vi "RSZVB Select PAE Measurement.vi"(6 "DUT Out (2)":i32=2, 7 "DUT In (1)":i32=1, 8 "error in (no error)":errorcluster {"code" format="%.0x"}, 9 "Trace Name (Trc1)":string="Trc1", 10 "Channel (1)":i32=1, 11 "VISA session":refnum<visa-resource-name>) -> (0 "error out":errorcluster {"code" format="%.0x"}, 3 "dup VISA session":refnum<visa-resource-name>)   [LabVIEW 2011]
doc: "This VI select the Power Added Efficiency (PAE) of an active 2-port device as measured quantity and to define the parameters for the PAE measurement. \n\nThe Power Added Efficiency (PAE) is the ratio of the added RF power generated by an active two-port device (e.g. an amplifier) to the supplied DC power PDC. The added RF power can be expressed as the difference between the power of the outgoing wave b2 at the output of the DUT and the power of the incident wave a1 at the input of the DUT.\n\nAssigns a measurement parameter to an existing trace or creates a trace and assigns a channel number, a name and a measurement parameter to it. The trace is not displayed.\n\nTo obtain reasonable results, the test model and the respective Constant must be selected in accordance to the test setup.\n\nRemote-control command(s):\nCALCulate<Ch>:PARameter:SDEFine '<string>', 'PAE21' | 'PAE12' | ...\nCALCulate<Ch>:PARameter:MEASure '<string>', 'PAE21' | 'PAE12' | ..."
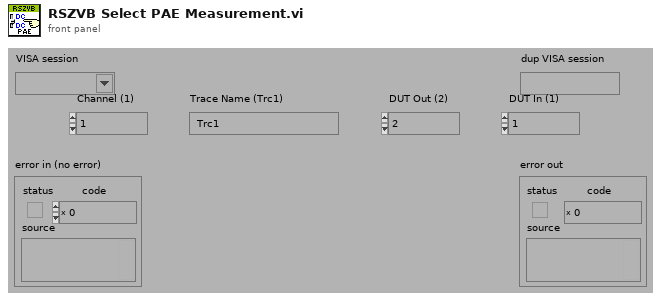
[diagram p1: front panel]
types:
  T1 = cluster{"Error Checking (T: On)":bool, "Installed Options":string[], "Data Valid?":bool, "Ports":i32, "Model":string[], "Option Checking (T: On)":bool}
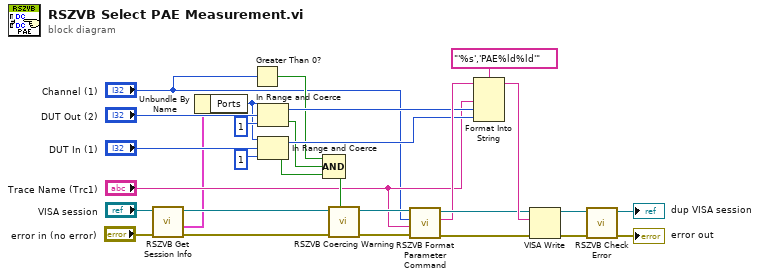
[diagram p0: block diagram]
diagram:
  n1 = call "RSZVB Get Session Info.vi"("error in (no error)"="error in (no error)", "VISA session"="VISA session") -> ("error out"=w4:errorcluster, "Session Info"=w2:T1, "dup VISA session"=w3:refnum<visa-resource-name>)  [unwired: 7 in]
  n2 = Unbundle By Name(w2) -> ("Ports"=w1:i32)
  n3 = Greater Than 0?(x="Channel (1)") -> (x > 0?=w16:bool)
  n4 = In Range and Coerce(upper limit=w1, x="DUT Out (2)", lower limit=1) -> (coerced(x)=w18:i32, In Range?=w15:bool)
  n5 = In Range and Coerce(upper limit=w1, x="DUT In (1)", lower limit=1) -> (coerced(x)=w17:i32, In Range?=w14:bool)
  n6 = Compound Arithmetic op=AND(w16, w15, w14) -> (w26:bool)
  n7 = call "RSZVB Coercing Warning.vi"("In Range?"=w26, "error in (no error)"=w4, "VISA session"=w3) -> ("error out"=w23:errorcluster, "dup VISA session"=w22:refnum<visa-resource-name>)  [unwired: 7 in]
  n8 = call "RSZVB Format Parameter Command.vi"("error in (no error)"=w23, "Trace Name (Trc1)"="Trace Name (Trc1)", "Channel (1)"="Channel (1)", "VISA session"=w22) -> ("error out"=w24:errorcluster, "Buffer"=w20:string, "dup VISA session"=w21:refnum<visa-resource-name>)  [unwired: 5 in]
  n9 = Format Into String(format string="'%s','PAE%ld%ld'", initial string=w20, "Trace Name (Trc1)", w18, w17) -> (resulting string=w25:string)  [unwired: 1 in, 1 out]
  n10 = VISA Write(VISA resource name=w21, write buffer=w25, error in (no error)=w24) -> (VISA resource name out=w27:refnum<visa-resource-name>, error out=w28:errorcluster)  [unwired: 1 out]
  n11 = call "RSZVB Check Error.vi"("error in (no error)"=w28, "VISA session"=w27) -> ("error out"=→"error out":errorcluster, "dup VISA session"=→"dup VISA session":refnum<visa-resource-name>)  [unwired: 8 in]
